vi "Generate Sine Sweep_v2.vi"() -> ()   [LabVIEW 2018]
uses:
  <vilib>/sound2/lvsound2.llb/Sound Data Format.ctl
  <vilib>/sound2/lvsound2.llb/Sampling Mode.ctl
  <vilib>/sound2/lvsound2.llb/Sound Output Write (DBL Single).vi
  <vilib>/addons/_NISVFA/_Generation/SoundVib_Generation.lvlib
panel:
  out "t":dbl
  in  "stop":bool
  out "error out":errorcluster
  in  "sound format":T1={"sample rate (S/s)"=44100.0, "number of channels"=1, "bits per sample"=16}
  in  "device ID":u32
  in  "chirp duration [s]":dbl=-1.0
  in  "sampling info":cluster{"Fs":dbl, "#s":u32}={"Fs"=44100.0, "#s"=1024} {"Fs" format="%.2p"}
  in  "frequency spacing":enum16{"Linear", "Logarithmic"}(ring)
  out "Waveform Graph":waveform(dbl)(graph)
  in  "frequency range [Hz]":cluster{"start":dbl, "stop":dbl}={"start"=20.0, "stop"=20000.0} {"stop" format="%.2f"; "start" format="%.2f"}
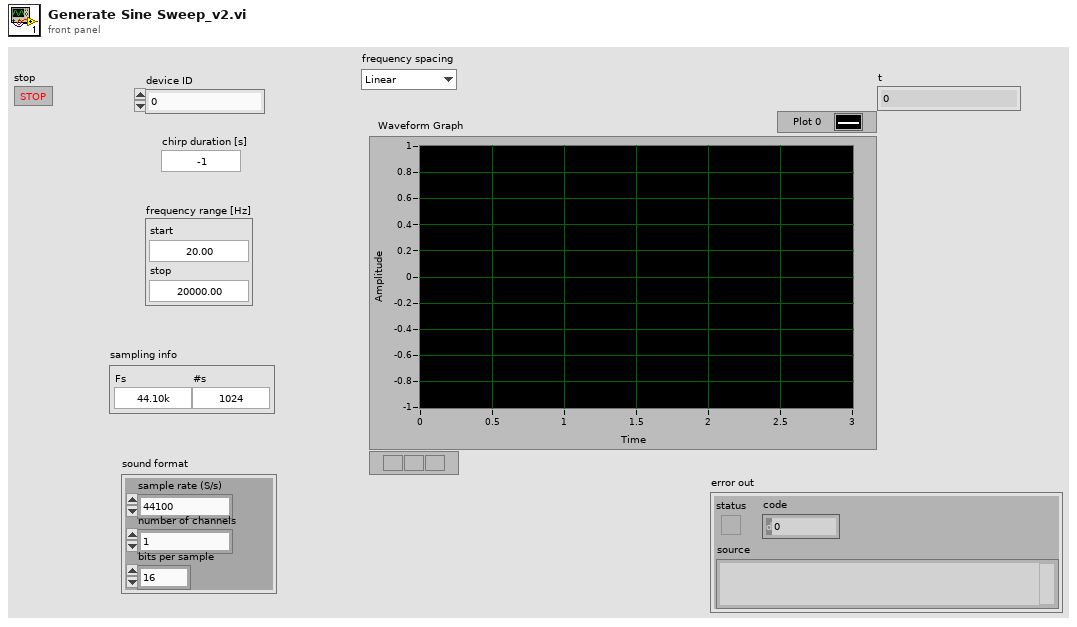
[diagram p1: front panel]
types:
  T1 = typedef "Sound Data Format.ctl" = cluster{"sample rate (S/s)":dbl, "number of channels":i32, "bits per sample":i32}
  T2 = typedef "Sampling Mode.ctl" = i32
  T3 = typedef "Sound Output Task ID.ctl" = u32
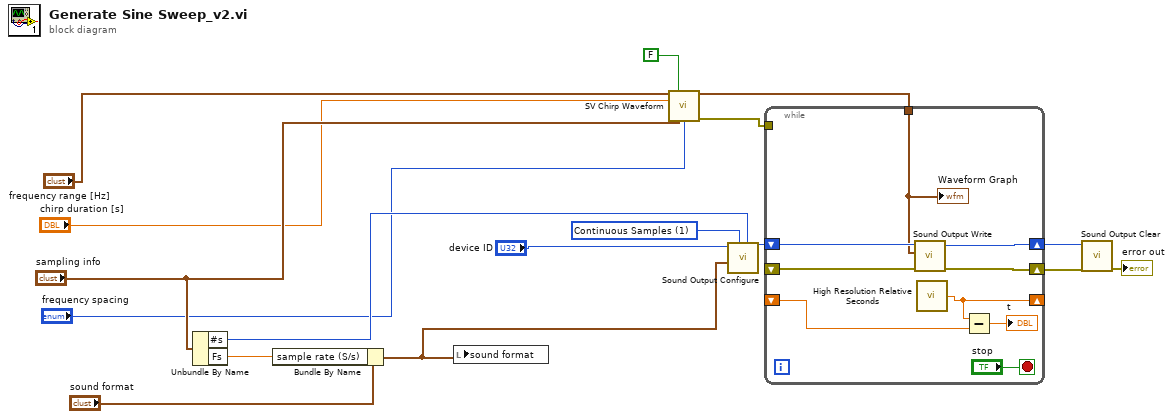
[diagram p0: block diagram]
diagram:
  w16 = T2 1 items=["Finite Samples", "Continuous Samples"] ("sample mode")
  n1 = Unbundle By Name("sampling info") -> ("#s"=w7:u32, "Fs"=w11:dbl)
  n2 = Bundle By Name(cluster="sound format", "sample rate (S/s)"=w11) -> (w13:T1)
  n3 = local write "sound format"(w13) -> ()
  n4 = call <vilib>:"SV Chirp Waveform.vi"("frequency range"="frequency range [Hz]", "reset signal (F)"=FALSE, "chirp duration [s]"="chirp duration [s]", "sampling info"="sampling info", "frequency spacing"="frequency spacing") -> ("chirp signal"=w3:waveform(dbl), "error out"=w2:errorcluster)  [unwired: 8 in, 1 out]
  n5 = call <vilib>:"Sound Output Configure.vi"("number of samples/ch"=w7, "sample mode"=w16, "sound format"=w13, "device ID"="device ID") -> ("task ID"=w10:T3)  [unwired: 6 in, 1 out]
  n6 = while {
    shift-right: [w25] -> w9
    shift-left: w10 -> [w26]
    shift-right: [w24] -> w8
    shift-left: _ -> [w18]
    shift-right: [w22] -> _
    shift-left: _ -> [w21]
    tunnel: w3 -> [w19]
    tunnel: w2 -> [_]
    stop <- "stop" stop-if-true
    n7 = call-poly <vilib>:"Sound Output Write.vi"("error in (no error)"=w18, "data"=w19, "task ID"=w26) -> ("error out"=w24:errorcluster, "task ID out"=w25:T3)  [unwired: 7 in]
    n8 = call <vilib>:"High Resolution Relative Seconds.vi"() -> ("relative seconds"=w22:dbl)
    n9 = Subtract(x=w22, y=w21) -> (x-y=→"t":dbl)
    "Waveform Graph" <- w19
  }
  n10 = call <vilib>:"Sound Output Clear.vi"("error in (no error)"=w8, "task ID"=w9) -> ("error out"=→"error out":errorcluster)  [unwired: 9 in]
